vi "B-Scan (Timed) DVR.vi"(9 "Scan definition":T2={"Max Scan Length"=0, "Update Rate"=1000, "Direction"=enum."Forwards"} {"Update Rate" format="%#_6f"; "Max Scan Length" format="%#_6f"}, 11 "scan data info":T4 {"Error Message" format="%04x"; "Message Header" format="%04x"; "IP"."MIP location" format="%#.0f"; "IP"."Location" format="%#.0f"; "PRF" format="%.0fHz"}) -> (0 "Update Display?":bool, 1 "B-Scan In Progress?":bool, 2 "B-Scan Index":i32, 3 "data value reference":refnum<data-value>)   [LabVIEW 2026, in "MicroPulse_Driver.lvlib"]
uses:
  MicroPulse_Driver.lvlib
  Data/Datatypes/MP - scan data info.ctl
  Data/Datatypes/MP - data output format.ctl
  Data/Datatypes/MP - retain scan.ctl
  Data/Datatypes/MP - axis positions (LLC).ctl
  Data/Datatypes/MP - fly scan range (timed).ctl
  Data/Datatypes/MP - inspection direction.ctl
  Low Level/FGV - B-Scan Active - Action [Enum].ctl
  <instrlib>/Micropulse/Micropulse.lvlib
panel:
  in  "X Scan definition":T1={"Max X Scan Length"=0, "Indexing\nResolution"=1000} {"Indexing\nResolution" format="%#_6f"; "Max X Scan Length" format="%#_6f"}
  # "X-Scan Index"
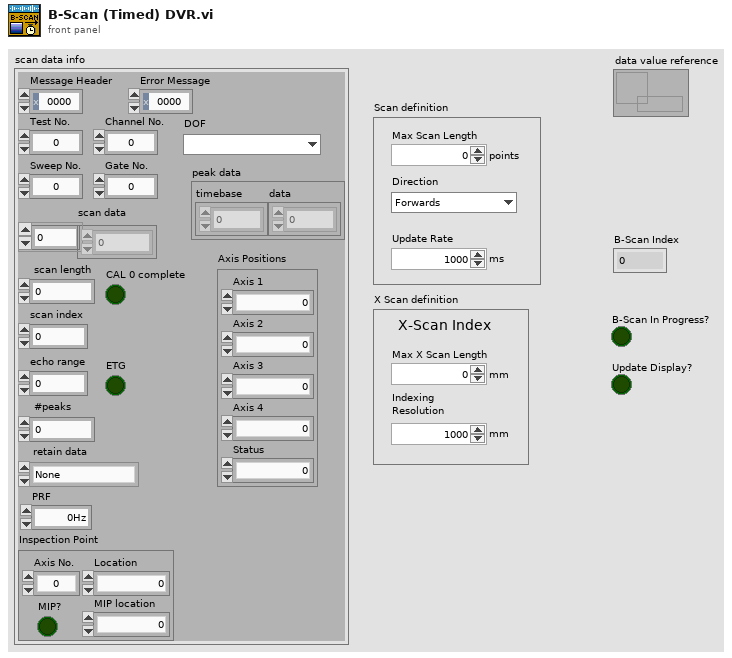
[diagram p1: front panel]
types:
  T1 = cluster{"Max X Scan Length":i32, "Indexing\nResolution":i32}
  T2 = typedef "Micropulse.lvlib/MP - fly scan range (timed).ctl" = cluster{"Max Scan Length":i32, "Update Rate":i32, "Direction":T3}
  T3 = typedef "Micropulse.lvlib/MP - inspection direction.ctl" = enum16{"Forwards", "Backwards"}
  T4 = typedef "Micropulse.lvlib/MP - scan data info.ctl" = cluster{"Message Header":u16, "Error Message":u16, "Test No.":u32, "Channel No.":u8, "Sweep No.":u32, "Gate No.":u32, "DOF":T5, "retain data":T6, "scan data":u16[], "scan length":i32, "scan index":i32, "peak data":cluster{"timebase":u16[], "data":u16[]}, "#peaks":i32, "PRF":dbl, "IP":cluster{"Axis No.":u8, "Location":u32, "MIP location":u32, "MIP?":bool}, "echo range":u16, "ETG":bool, "CAL 0 complete":bool, "Axis Positions":T7}
  T5 = typedef "Micropulse.lvlib/MP - data output format.ctl" = enum16{"", "8-bit Mode", "10-bit Mode", "12-bit Mode", "16-bit Mode", "8-bit Log Mode", "12-bit Packed Mode"}
  T6 = typedef "Micropulse.lvlib/MP - retain scan.ctl" = enum16{"None", "Ascan", "Peaks"}
  T7 = typedef "Micropulse.lvlib/MP - axis positions (LLC).ctl" = cluster{"Axis 1":u32, "Axis 2":u32, "Axis 3":u32, "Axis 4":u32, "Status":u8}
  T8 = typedef "MicroPulse_Driver.lvlib/FGV - B-Scan Active - Action [Enum].ctl" = enum16{"Read", "Read & Reset Start Flag", "Start B-Scan", "B-Scan Finished"}
  T9 = cluster{"Lowest location":i32, "Highest location":i32}
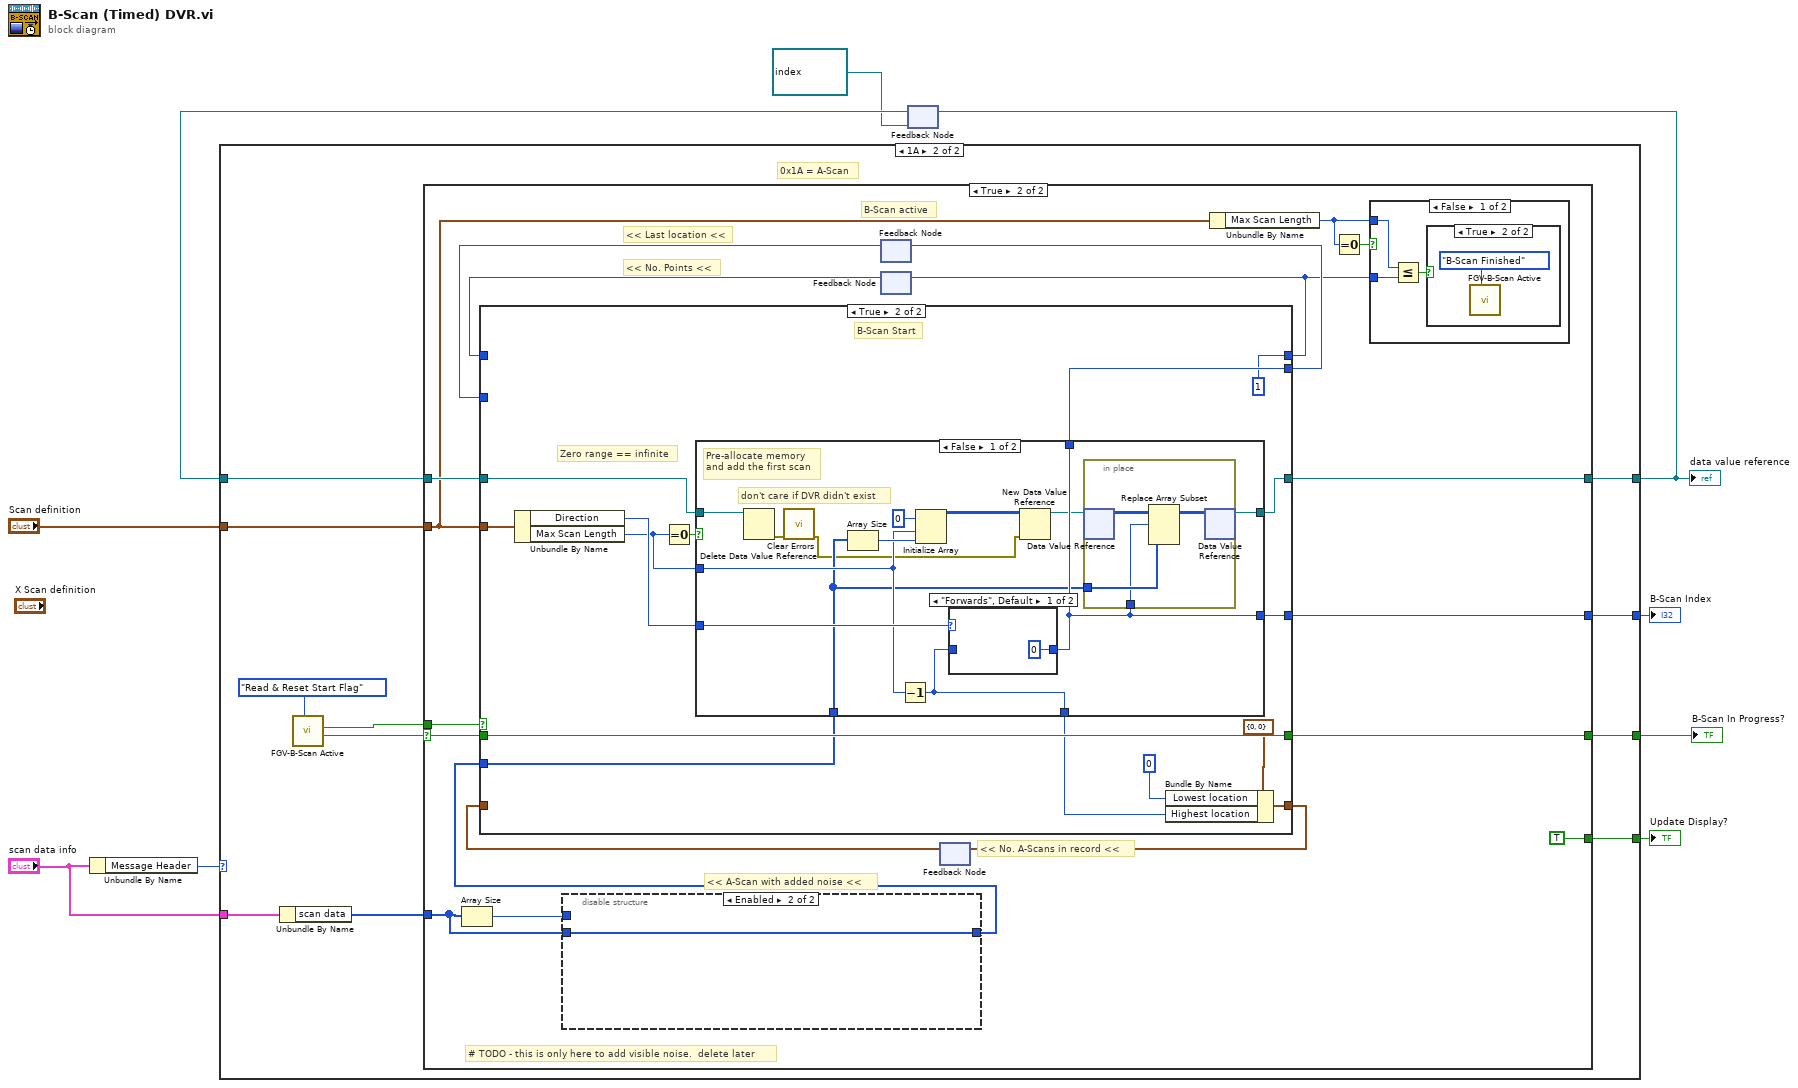
[diagram p0: block diagram]
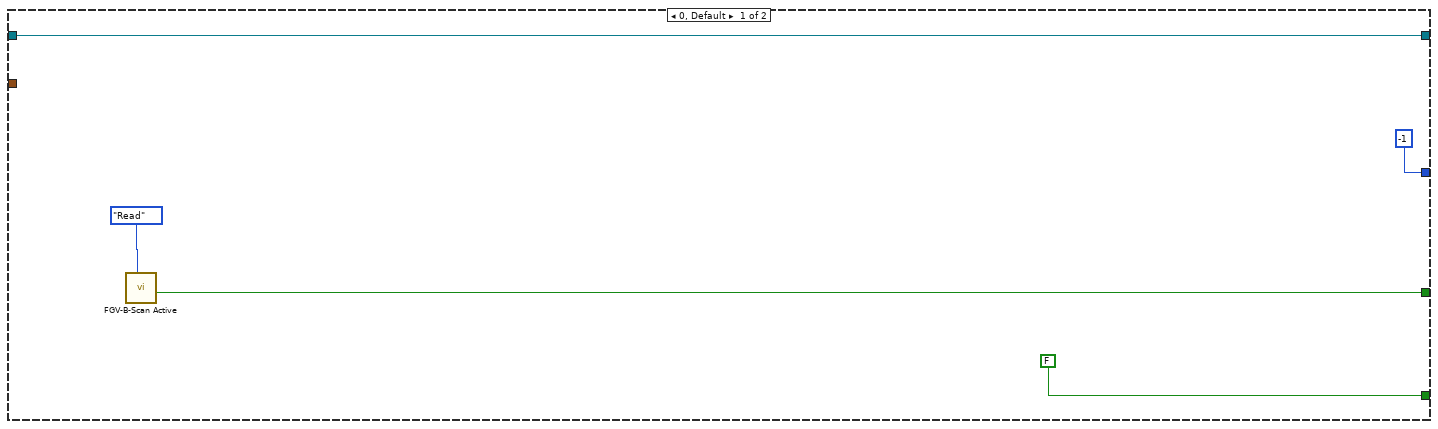
[diagram p2: hidden frame]
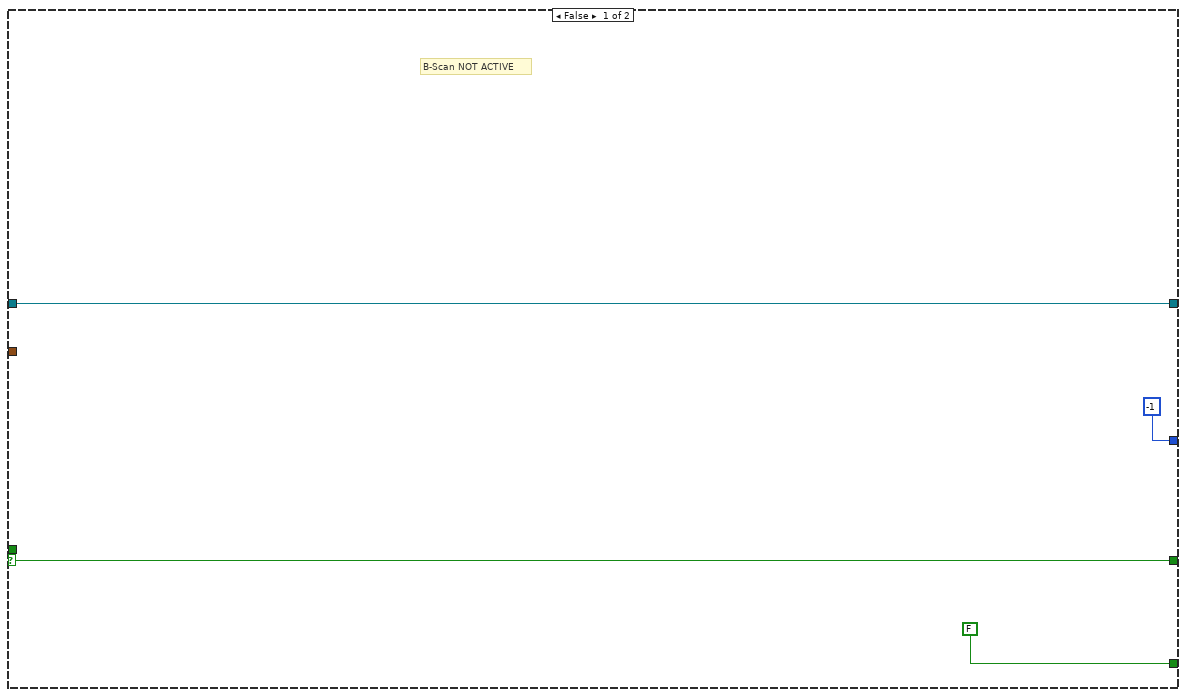
[diagram p3: hidden frame]
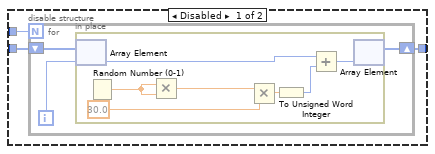
[diagram p4: hidden frame]
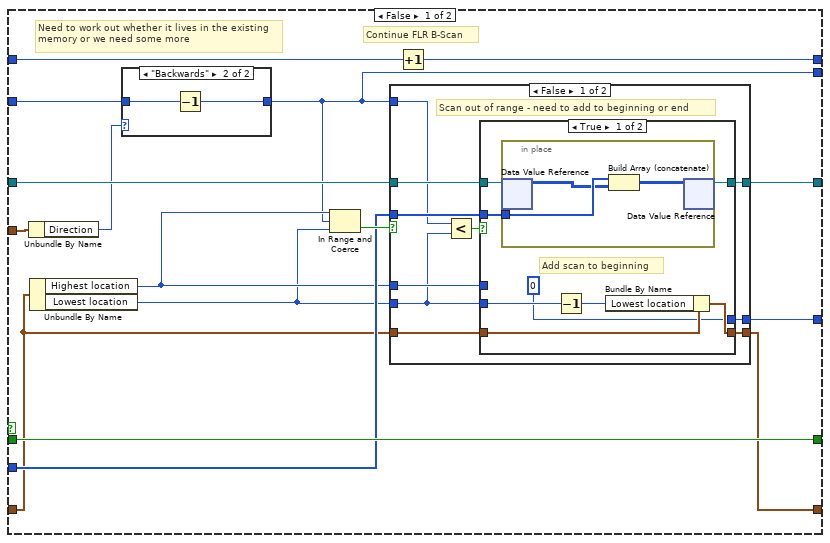
[diagram p7: hidden frame]
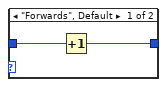
[diagram p8: hidden frame]
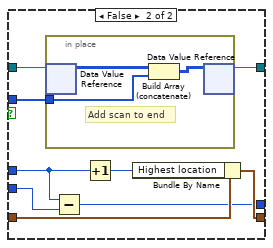
[diagram p9: hidden frame]
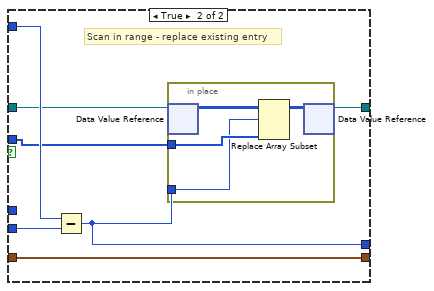
[diagram p10: hidden frame]
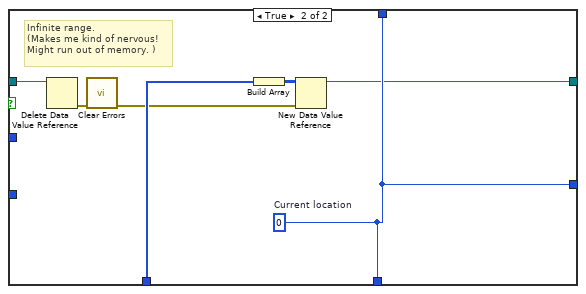
[diagram p12: hidden frame]
diagram:
  n1 = Unbundle By Name("scan data info") -> ("Message Header"=w9:u16)
  n2 = feedback #1(refnum<data-value> refnum ("data value reference")) -> (w6:refnum<data-value>)
  n3 = case shown="1A" w9 {
    tunnel: "scan data info" -> [_ w25]
    tunnel: "Scan definition" -> [_ w19]
    tunnel: [w14 w23] -> w7
    tunnel: w6 -> [w14 w22]
    tunnel: [w11 w21] -> w5
    tunnel: [FALSE w20] -> w4
    tunnel: [-1 ("Current location") w15] -> w2
    frame 0, Default {
      n4 = call "FGV-B-Scan Active.vi"("Action"=FGV_-_B-Scan_Active_-_Action_[Enum]."Read") -> ("B-Scan In Progress?"=w11:bool)  [unwired: 8 in, 2 out]
    }
    frame 26 {
      # "0x1A = A-Scan"
      n5 = Unbundle By Name(w25) -> ("scan data"=w24:u16[])
      n6 = call "FGV-B-Scan Active.vi"("Action"=FGV_-_B-Scan_Active_-_Action_[Enum]."Read & Reset Start Flag") -> ("B-Scan In Progress?"=w16:bool, "B-Scan Start?"=w17:bool)  [unwired: 8 in, 1 out]
      n7 = case shown="True" w16 {
        selector: w16 -> [w28 w44]
        tunnel: w17 -> [_ w47]
        tunnel: w22 -> [w29 w48]
        tunnel: [w29 w41] -> w23
        tunnel: w24 -> [_ w40]
        tunnel: w19 -> [_ w34]
        tunnel: [w28 w45] -> w21
        tunnel: [FALSE TRUE] -> w20
        tunnel: [-1 ("Current location") w30] -> w15
        frame False {
          # "B-Scan NOT ACTIVE"
        }
        frame True {
          # "<< No. Points <<"
          # "<< Last location <<"
          # "<< A-Scan with added noise <<"
          # "B-Scan active"
          # "<< No. A-Scans in record <<"
          # "# TODO - this is only here to add visible noise.  delete later"
          n8 = Array Size(array=w40) -> (size(s)=w42:i32)
          n9 = disable-structure shown="Enabled" {
            disable-tunnel: w42 -> [w51 _]
            disable-tunnel: w40 -> [w50 w62]
            disable-tunnel: [w49 w62] -> w39
            frame Disabled {
              n10 = for {
                N: w51 -> [_]
                shift-right: [w52] -> w49
                shift-left: w50 -> [w54]
                i -> [w53]
                n11 = in-place {
                  n12 = in-place-array #2(w54, w53) -> (w58:u16)
                  n13 = Random Number (0-1)() -> (number: 0 to 1=w55:dbl)
                  n14 = Multiply(x=w55, y=w55) -> (x*y=w56:dbl)
                  n15 = Multiply(x=w56, y=30.0) -> (x*y=w60:dbl)
                  n16 = To Unsigned Word Integer(number=w60) -> (unsigned 16bit integer=w59:u16)
                  n17 = Add(x=w58, y=w59) -> (x+y=w57:u16)
                  n18 = in-place-array #2(w57) -> (w52:u16[])  [unwired: 1 out]
                }
              }
            }
            frame Enabled {
            }
          }
          n19 = feedback #3() -> (w36:i32)  [unwired: 1 in]
          n20 = feedback #4() -> (w35:i32)  [unwired: 1 in]
          n21 = feedback #5() -> (w46:T9)  [unwired: 1 in]
          n22 = case shown="True" w47 {
            tunnel: w48 -> [w82 w131]
            tunnel: [w80 w145] -> w41
            tunnel: w34 -> [w73 w144]
            tunnel: w36 -> [w71 _]
            tunnel: w46 -> [w75 _]
            tunnel: [w81 w143] -> w45
            tunnel: w44 -> [w81 w143]
            tunnel: w39 -> [w78 w142]
            tunnel: [w74 w140] -> w38
            tunnel: [w70 w134] -> w37
            tunnel: [w68 1 ("Current location")] -> w31
            tunnel: w35 -> [w69 _]
            tunnel: [w67 w132] -> w30
            frame False {
              # "Continue FLR B-Scan"
              # "Need to work out whether it lives in the existing memory or we need some more"
              n23 = Unbundle By Name(w73) -> ("Direction"=w72:T3)
              n24 = Unbundle By Name(w75) -> ("Highest location"=w77:i32, "Lowest location"=w76:i32)
              n25 = case shown="\"Backwards\"" w72 {
                tunnel: w71 -> [w84 w86]
                tunnel: [w83 w85] -> w70
                frame "Forwards", Default {
                  n26 = Increment(x=w84) -> (x+1=w83:i32)
                }
                frame "Backwards" {
                  n27 = Decrement(x=w86) -> (x-1=w85:i32)
                }
              }
              n28 = In Range and Coerce(upper limit=w77, x=w70, lower limit=w76) -> (In Range?=w79:bool)  [unwired: 1 out]
              n29 = case shown="False" w79 {
                tunnel: w82 -> [w96 w122]
                tunnel: [w95 w123] -> w80
                tunnel: w70 -> [w93 w126]
                tunnel: w78 -> [w94 w120]
                tunnel: w77 -> [w91 _]
                tunnel: w76 -> [w88 w124]
                tunnel: w75 -> [w90 w125]
                tunnel: [w89 w125] -> w74
                tunnel: [w87 w121] -> w67
                frame False {
                  # "Scan out of range - need to add to beginning or end"
                  n30 = Less?(x=w93, y=w88) -> (x < y?=w92:bool)
                  n31 = case shown="True" w92 {
                    tunnel: w96 -> [w98 w110]
                    tunnel: [w99 w108] -> w95
                    tunnel: w94 -> [w97 w109]
                    tunnel: w91 -> [_ w113]
                    tunnel: w88 -> [w103 w112]
                    tunnel: w90 -> [w104 w116]
                    tunnel: [w101 w114] -> w89
                    tunnel: [0 w111] -> w87
                    frame True {
                      # "Add scan to beginning"
                      n32 = in-place {
                        in-place-border: w97 -> [w107]
                        n33 = in-place-dvr #6(w98) -> (w106:u16[][])  [unwired: 1 out]
                        n34 = Build Array (concatenate)(w107, w106) -> (w105:u16[][])
                        n35 = in-place-dvr #6(w105) -> (w99:refnum<data-value>)  [unwired: 1 out]
                      }
                      n36 = Decrement(x=w103) -> (x-1=w102:i32)
                      n37 = Bundle By Name(cluster=w104, "Lowest location"=w102) -> (w101:T9)
                    }
                    frame False {
                      n38 = in-place {
                        in-place-border: w109 -> [w119]
                        # "Add scan to end"
                        n39 = in-place-dvr #7(w110) -> (w117:u16[][])  [unwired: 1 out]
                        n40 = Build Array (concatenate)(w117, w119) -> (w118:u16[][])
                        n41 = in-place-dvr #7(w118) -> (w108:refnum<data-value>)  [unwired: 1 out]
                      }
                      n42 = Subtract(x=w113, y=w112) -> (x-y=w111:i32)
                      n43 = Increment(x=w113) -> (x+1=w115:i32)
                      n44 = Bundle By Name(cluster=w116, "Highest location"=w115) -> (w114:T9)
                    }
                  }
                }
                frame True {
                  # "Scan in range - replace existing entry"
                  n45 = Subtract(x=w126, y=w124) -> (x-y=w121:i32)
                  n46 = in-place {
                    in-place-border: w120 -> [w130]
                    in-place-border: w121 -> [w129]
                    n47 = in-place-dvr #8(w122) -> (w127:u16[][])  [unwired: 1 out]
                    n48 = Replace Array Subset(array=w127, new element=w130, index (row)=w129) -> (w128:u16[][])  [unwired: 1 in]
                    n49 = in-place-dvr #8(w128) -> (w123:refnum<data-value>)  [unwired: 1 out]
                  }
                }
              }
              n50 = Increment(x=w69) -> (x+1=w68:i32)
            }
            frame True {
              # "Zero range == infinite"
              # "B-Scan Start"
              n51 = Unbundle By Name(w144) -> ("Direction"=w139:T3, "Max Scan Length"=w136:i32)
              n52 = Equal To 0?(x=w136) -> (x = 0?=w137:bool)
              n53 = case shown="False" w137 {
                tunnel: [w148 w165] -> w145
                tunnel: w136 -> [w155 _]
                tunnel: w142 -> [w147 w171]
                tunnel: w139 -> [w156 _]
                tunnel: [w154 w170] -> w138
                tunnel: [w151 w170] -> w134
                tunnel: [w151 w170] -> w132
                tunnel: w131 -> [w152 w167]
                frame False {
                  # "don't care if DVR didn't exist"
                  # "Pre-allocate memory\nand add the first scan"
                  n54 = Delete Data Value Reference(data value reference=w152) -> (error out=w153:errorcluster)  [unwired: 1 in, 1 out]
                  n55 = call <vilib>:"Clear Errors.vi"("error in (no error)"=w153) -> ("error out"=w146:errorcluster)  [unwired: 5 in, 1 out]
                  n56 = Array Size(array=w147) -> (size(s)=w157:i32)
                  n57 = Decrement(x=w155) -> (x-1=w154:i32)
                  n58 = Initialize Array(u16 0 ("index"), w155, w157) -> (w149:u16[][])
                  n59 = case shown="\"Forwards\", Default" w156 {
                    tunnel: w154 -> [_ w164]
                    tunnel: [0 w164] -> w151
                    frame "Forwards", Default {
                    }
                    frame "Backwards" {
                    }
                  }
                  n60 = New Data Value Reference(data value=w149, error in=w146) -> (data value reference=w150:refnum<data-value>)  [unwired: 1 out]
                  n61 = in-place {
                    in-place-border: w147 -> [w162]
                    in-place-border: w151 -> [w161]
                    n62 = in-place-dvr #9(w150) -> (w160:u16[][])  [unwired: 1 out]
                    n63 = Replace Array Subset(array=w160, new element=w162, index (row)=w161) -> (w159:u16[][])  [unwired: 1 in]
                    n64 = in-place-dvr #9(w159) -> (w148:refnum<data-value>)  [unwired: 1 out]
                  }
                }
                frame True {
                  w170 = 0  # Current location
                  # "Infinite range.\n(Makes me kind of nervous!\nMight run out of memory. )"
                  n65 = Delete Data Value Reference(data value reference=w167) -> (error out=w168:errorcluster)  [unwired: 1 in, 1 out]
                  n66 = call <vilib>:"Clear Errors.vi"("error in (no error)"=w168) -> ("error out"=w169:errorcluster)  [unwired: 5 in, 1 out]
                  n67 = Build Array(w171) -> (w166:u16[][])
                  n68 = New Data Value Reference(data value=w166, error in=w169) -> (data value reference=w165:refnum<data-value>)  [unwired: 1 out]
                }
              }
              n69 = Bundle By Name(cluster=T9 {"Lowest location"=0, "Highest location"=0} ("input cluster"), "Lowest location"=0, "Highest location"=w138) -> (w140:T9)
            }
          }
          n70 = feedback-in #3(w37) -> ()
          n71 = feedback-in #4(w31) -> ()
          n72 = feedback-in #5(w38) -> ()
          n73 = Unbundle By Name(w34) -> ("Max Scan Length"=w32:i32)
          n74 = Equal To 0?(x=w32) -> (x = 0?=w33:bool)
          n75 = case shown="False" w33 {
            tunnel: w32 -> [w64 _]
            tunnel: w31 -> [w65 _]
            frame False {
              n76 = Less Or Equal?(x=w64, y=w65) -> (x <= y?=w63:bool)
              n77 = case shown="True" w63 {
                frame False {
                }
                frame True {
                  n78 = call "FGV-B-Scan Active.vi"("Action"=FGV_-_B-Scan_Active_-_Action_[Enum]."B-Scan Finished") -> ()  [unwired: 8 in, 3 out]
                }
              }
            }
            frame True {
              # "Do nothing\ninfinite scan"
            }
          }
        }
      }
    }
  }
  "data value reference" <- w7
  "Update Display?" <- w4
  "B-Scan In Progress?" <- w5
  "B-Scan Index" <- w2
  n79 = feedback-in #1(w7) -> ()
